vi "GLIMPSE window average.vi"(4 "error in (no error)":errorcluster) -> (0 "error out":errorcluster)   [LabVIEW 2011]
doc: "Performs a (non-destructive) jumping or sliding average of frames in an acquisition file and stores the result in a new acquisition file."
uses:
  Seq file v 1/Offset table.ctl
  Seq file v 1/Offset.ctl
  Seq file v 1/file number.ctl
  GLIMPSE Globals.vi
panel:
  in  "Window type":enum16{"Sliding", "Jumping"}(ring)
  in  "Input from existing":path=path "d:/1.glimpse"
  in  "Output to new directory":path=path "d:/1.glimpse"
  out "Progress":i16(slide) scale=1.0..100.0
  in  "Abort":bool
  in  "Frames to average":u32=8
  in  "Go ahead":bool
  # "This VI does not create header2 data."
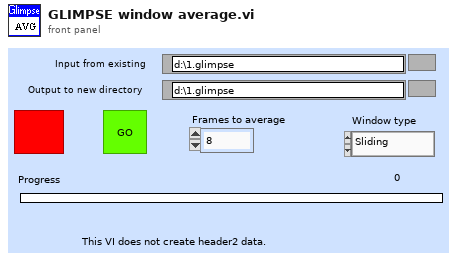
[diagram p1: front panel]
types:
  T1 = typedef "Header2 file data.ctl" = cluster{"Camera":string, "Microscope":string, "Microscope software version":string, "Laser names":string[], "Filter names":string[], "Lasers array":u16[][], "Filter array":u16[], "Flow rate array":dbl[], "Temperature array":dbl[], "Field array":u16[], "Is header2 info present?":bool, "Description Info":string, "Stage xyz array":dbl[][]}
  T2 = typedef "Header file data.ctl" = cluster{"Frames Acquired":u32, "Region width":i32, "Region height":i32, "Element 0 of TTB":u32, "time of 1st frame, \nsec since 1/1/04":dbl, "TTB Array (ms)":u32[], "Offsets Array":T3, "Pixel depth":u32}
  T3 = typedef "Offset table.ctl" = cluster{"offset":T4, "file number":T5}[]
  T4 = typedef "Offset.ctl" = i32
  T5 = typedef "file number.ctl" = u8
  T6 = typedef "Sequence files handle.ctt" = cluster{"Sequence files directory path":path, "Sequence files refnum array":refnum<file>[]}
  T7 = typedef "IMAQ Image.ctl" = refnum<image>
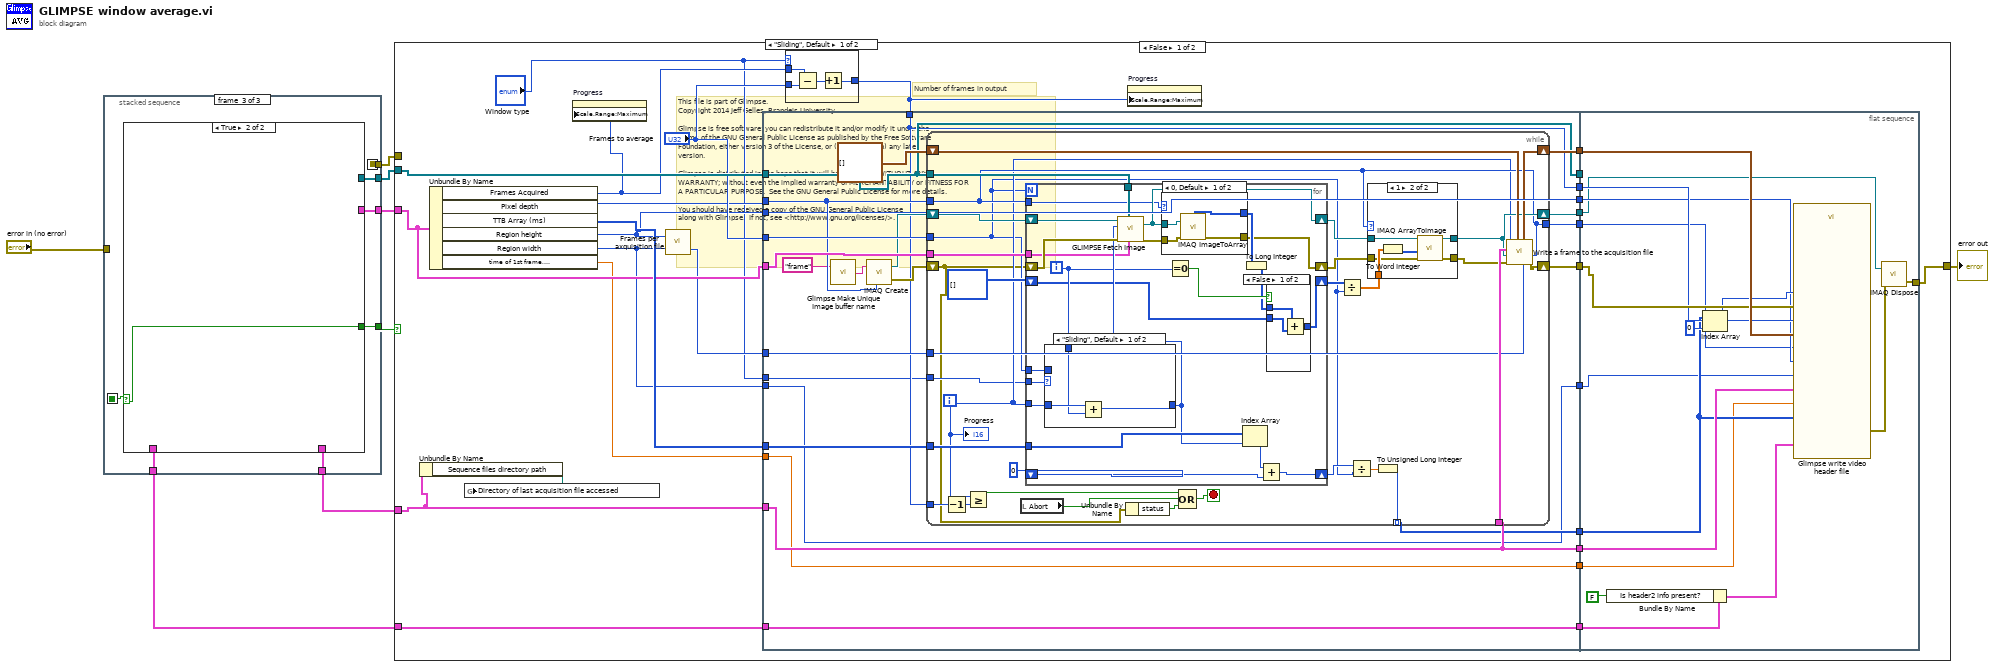
[diagram p0: block diagram]
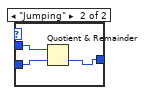
[diagram p2: hidden frame]
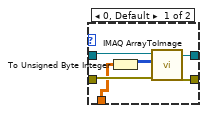
[diagram p3: hidden frame]
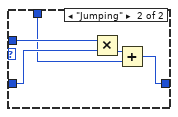
[diagram p4: hidden frame]
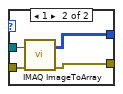
[diagram p6: hidden frame]
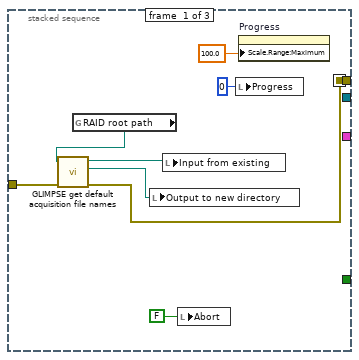
[diagram p8: hidden frame]
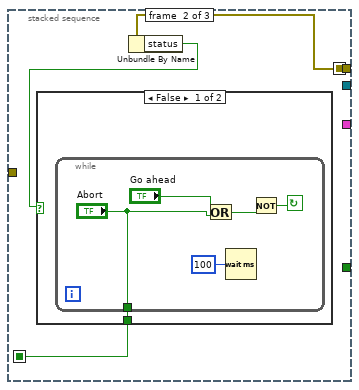
[diagram p9: hidden frame]
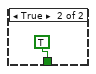
[diagram p10: hidden frame]
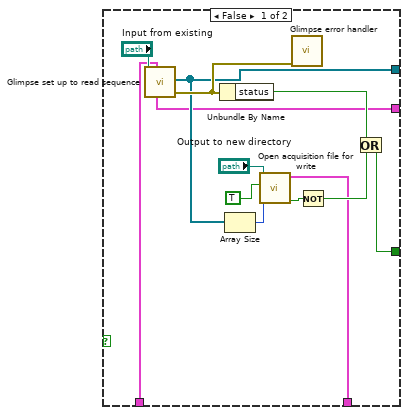
[diagram p11: hidden frame]
diagram:
  # "This file is part of Glimpse. \nCopyright 2014 Jeff Gelles, Brandeis University.    \n\nGlimpse is free software: you can redistribute it and/or modify it under the \nterms of the GNU General Public License as published by the Free Software \nFoundation, either version 3 of the License, or (at your option) any later \nversion.\n\nGlimpse is distributed in the hope that it will be useful, but WITHOUT ANY \nWARRANTY; without even the implied warranty of MERCHANTABILITY or FITNESS FOR \nA PARTICULAR PURPOSE.  See the GNU General Public License for more details.\n\nYou should have received a copy of the GNU General Public License\nalong with Glimpse.  If not, see <http://www.gnu.org/licenses/>."
  n1 = stacked-sequence {
    seq-local: [w11 _ _] -> [_ w19 w29]
    seq-local: [_ w17 _] -> [_ _ w33]
    tunnel: "error in (no error)" -> [w14 _ _]
    tunnel: [_ _ w32] -> w7
    tunnel: [_ _ w31] -> w6
    tunnel: [_ _ w30] -> w5
    tunnel: [_ _ w29] -> w3
    tunnel: [_ _ w28] -> w2
    tunnel: [_ _ w27] -> w1
    frame #0 {
      n2 = global read "GLIMPSE Globals.vi" "RAID root path"() -> (w15:path)
      n3 = call "GLIMPSE get default acquisition file names.vi"("error in"=w14, "RAID root path"=w15) -> ("error out"=w11:errorcluster, "next directory path"=w13:path, "last directory path"=w12:path)  [unwired: 5 out]
      n4 = local write "Output to new directory"(w13) -> ()
      n5 = local write "Input from existing"(w12) -> ()
      n6 = local write "Abort"(FALSE ("Abort")) -> ()
      n7 = local write "Progress"(i16 0 ("Progress")) -> ()
      n8 = property on="Progress" class="Slide (strict)"("Scale.Range:Maximum"=100.0) -> ()  [unwired: 2 in, 2 out]
    }
    frame #1 {
      n9 = Unbundle By Name(w19) -> ("status"=w18:bool)
      n10 = case shown="False" w18 {
        tunnel: [w20 TRUE ("Abort")] -> w17
        frame False {
          n11 = while {
            tunnel: ["Abort"] -> w20
            stop <- w25 continue-if-true
            n12 = Or(x="Go ahead", y="Abort") -> (x .or. y?=w23:bool)
            n13 = Wait (ms)(milliseconds to wait=u32 100) -> ()  [unwired: 1 out]
            n14 = Not(x=w23) -> (.not. x?=w25:bool)
          }
        }
        frame True {
        }
      }
    }
    frame #2 {
      n15 = case shown="True" w33 {
        selector: w33 -> [_ w47]
        tunnel: [w40 w47] -> w32
        tunnel: [w38 _] -> w31
        tunnel: [w36 _] -> w30
        tunnel: [w35 _] -> w28
        tunnel: [w34 _] -> w27
        frame False {
          n16 = call "Glimpse set up to read sequence.vi"("acquisition directory path"="Input from existing") -> ("Header2 file data out"=w34:T1, "Header file data out"=w35:T2, "Acquisition refnum array"=w36:refnum<file>[], "error out"=w39:errorcluster)  [unwired: 1 in, 2 out]
          n17 = Unbundle By Name(w39) -> ("status"=w42:bool)
          n18 = Array Size(array=w36) -> (size(s)=w37:i32)
          n19 = call "Open acquisition file for write.vi"("Number of acquisition files"=w37, "Use new?"=TRUE, "New directory to create"="Output to new directory") -> ("OK?"=w43:bool, "Sequence files handle"=w38:T6)  [unwired: 1 in, 5 out]
          n20 = call "Glimpse error handler.vi"("error in"=w39) -> ()  [unwired: 1 in, 6 out]
          n21 = Not(x=w43) -> (.not. x?=w41:bool)
          n22 = Or(x=w42, y=w41) -> (x .or. y?=w40:bool)
        }
        frame True {
        }
      }
    }
  }
  n23 = case shown="False" w7 {
    tunnel: w6 -> [w51 _]
    tunnel: w5 -> [w75 _]
    tunnel: [w74 w210] -> w4
    tunnel: w3 -> [_ w210]
    tunnel: w2 -> [w69 _]
    tunnel: w1 -> [w49 _]
    frame False {
      # "Number of frames in output"
      n24 = Unbundle By Name(w51) -> ("Sequence files directory path"=w50:path)
      n25 = Unbundle By Name(w69) -> ("Frames Acquired"=w64:u32, "Pixel depth"=w71:u32, "TTB Array (ms)"=w70:u32[], "Region height"=w66:i32, "Region width"=w67:i32, "time of 1st frame, \nsec since 1/1/04"=w65:dbl)
      n26 = global write "GLIMPSE Globals.vi" "Directory of last acquisition file accessed"(w50) -> ()
      n27 = property on="Progress" class="Slide (strict)"("Scale.Range:Maximum"=w64) -> ()  [unwired: 2 in, 2 out]
      n28 = call "Frames per axquisition file.vi"("Output frame width"=w67, "Output frame height"=w66) -> ("Frames per acquisition file"=w68:i32)  [unwired: 1 out]
      n29 = flat-sequence {
        tunnel: "Frames to average" -> [w104]
        tunnel: w51 -> [w100]
        tunnel: [w100] -> w63
        tunnel: w75 -> [w99]
        tunnel: [w99] -> w62
        tunnel: w72 -> [w85]
        tunnel: [w85] -> w61
        tunnel: w71 -> [w94]
        tunnel: w70 -> [w97]
        tunnel: w69 -> [w96]
        tunnel: w68 -> [w95]
        tunnel: w67 -> [w89]
        tunnel: [w89] -> w60
        tunnel: w66 -> [w88]
        tunnel: [w88] -> w59
        tunnel: w65 -> [w87]
        tunnel: [w87] -> w58
        tunnel: [w102] -> w57
        tunnel: [w101] -> w56
        tunnel: [w98] -> w55
        tunnel: [w90] -> w54
        tunnel: [w86] -> w53
        tunnel: "Window type" -> [w84]
        tunnel: w49 -> [w83]
        tunnel: [w83] -> w48
        tunnel: w63 -> [w207]
        tunnel: w62 -> [w205]
        tunnel: [w194] -> w74
        tunnel: w61 -> [w204]
        tunnel: w53 -> [w198]
        tunnel: w60 -> [w200]
        tunnel: w59 -> [w199]
        tunnel: w58 -> [w197]
        tunnel: w57 -> [w208]
        tunnel: w56 -> [w206]
        tunnel: w55 -> [w202]
        tunnel: w54 -> [w196]
        tunnel: w48 -> [w193]
        frame #0 {
          n30 = call "Glimpse Make Unique Image buffer name.vi"("Buffer  base name"="frame" ("Image Name")) -> ("Image Name"=w92:string)  [unwired: 1 out]
          n31 = call "IMAQ Create"("Image Name"=w92, "Image Type"=w94) -> ("New Image"=w93:T7, "error out"=w105:errorcluster)  [unwired: 2 in, 1 out]
          n32 = while {
            tunnel: w104 -> [w108]
            shift-right: [w130] -> w101
            shift-left: w105 -> [w106]
            tunnel: w97 -> [w135]
            tunnel: [w132] -> w98 mode=indexing
            shift-right: [w129] -> w102
            shift-left: T3 [] ("Offset table out") -> [w128]
            tunnel: w100 -> [w127]
            tunnel: w99 -> [w126]
            tunnel: w94 -> [w116]
            tunnel: w96 -> [w125]
            tunnel: w95 -> [w124]
            shift-right: [w117] -> w90
            shift-left: w93 -> [w131]
            tunnel: [w116] -> w86
            tunnel: w85 -> [w113]
            tunnel: w84 -> [w109]
            i -> [w115]
            stop <- w111 stop-if-true
            n33 = Decrement(x=w113) -> (x-1=w114:u32)
            n34 = Greater Or Equal?(x=w115, y=w114) -> (x >= y?=w112:bool)
            n35 = local read "Abort"() -> (w110:bool)
            n36 = for {
              N: w108 -> [_]
              tunnel: w115 -> [w170]
              shift-right: [w154] -> w120
              shift-left: w106 -> [w164]
              shift-right: [w169] -> w134
              shift-left: 0 -> [w168]
              tunnel: w135 -> [w166]
              tunnel: w126 -> [w162]
              tunnel: w125 -> [w161]
              tunnel: w116 -> [w152]
              shift-right: [w153] -> w119
              shift-left: w131 -> [w165]
              shift-right: [w155] -> w122
              shift-left: i32[][] [] -> [w157]
              tunnel: w109 -> [w151]
              tunnel: w108 -> [w150]
              i -> [w158]
              n37 = case shown="\"Sliding\", Default" w151 {
                tunnel: w170 -> [w173 w177]
                tunnel: [w172 w174] -> w163
                tunnel: w158 -> [w171 w175]
                tunnel: w150 -> [_ w178]
                frame "Sliding", Default {
                  n38 = Add(x=w173, y=w171) -> (x+y=w172:i32)
                }
                frame "Jumping" {
                  n39 = Multiply(x=w178, y=w177) -> (x*y=w176:u32)
                  n40 = Add(x=w176, y=w175) -> (x+y=w174:u32)
                }
              }
              n41 = call "GLIMPSE Fetch Image.vi"("Header file data"=w161, "Acqisition files refnums"=w162, "error in"=w164, "Logical Frame Number\n(starting with zero)"=w163, "Image In"=w165) -> ("error out"=w160:errorcluster, "Image Out"=w153:T7)  [unwired: 2 in, 3 out]
              n42 = case shown="0, Default" w152 {
                tunnel: w153 -> [w185 w190]
                tunnel: w160 -> [w186 w189]
                tunnel: [w183 w187] -> w156
                tunnel: [w184 w188] -> w154
                frame 0, Default {
                  n43 = call "IMAQ ImageToArray"("error in (no error)"=w186, "Image"=w185) -> ("error out"=w184:errorcluster, "Image Pixels (U8)"=w183:u8[][])  [unwired: 1 in, 4 out]
                }
                frame 1 {
                  n44 = call "IMAQ ImageToArray"("error in (no error)"=w189, "Image"=w190) -> ("error out"=w188:errorcluster, "Image Pixels (I16)"=w187:i16[][])  [unwired: 1 in, 4 out]
                }
              }
              n45 = Equal To 0?(x=w158) -> (x = 0?=w159:bool)
              n46 = Index Array(array=w166, index=w163) -> (element=w167:u32)
              n47 = To Long Integer(number=w156) -> (32bit integer=w149:i32[][])
              n48 = Add(x=w167, y=w168) -> (x+y=w169:u32)
              n49 = case shown="False" w159 {
                tunnel: w157 -> [w180 _]
                tunnel: [w179 w182] -> w155
                tunnel: w149 -> [w181 w182]
                frame False {
                  n50 = Add(x=w181, y=w180) -> (x+y=w179:i32[][])
                }
                frame True {
                }
              }
            }
            n51 = Unbundle By Name(w106) -> ("status"=w107:bool)
            n52 = Compound Arithmetic op=OR(w112, w110, w107) -> (w111:bool)
            n53 = Divide(x=w122, y=w108) -> (x/y=w121:dbl[][])
            n54 = Divide(x=w134, y=w108) -> (x/y=w133:dbl)
            n55 = case shown="1" w116 {
              tunnel: w121 -> [w137 w147]
              tunnel: w120 -> [w139 w146]
              tunnel: w119 -> [w140 w145]
              tunnel: [w141 w144] -> w117
              tunnel: [w142 w143] -> w118
              frame 0, Default {
                n56 = To Unsigned Byte Integer(number=w137) -> (unsigned 8bit integer=w138:u8[][])
                n57 = call "IMAQ ArrayToImage"("error in (no error)"=w139, "Image Pixels (U8)"=w138, "Image"=w140) -> ("error out"=w142:errorcluster, "Image Out"=w141:T7)  [unwired: 3 in, 4 out]
              }
              frame 1 {
                n58 = To Word Integer(number=w147) -> (16bit integer=w148:i16[][])
                n59 = call "IMAQ ArrayToImage"("error in (no error)"=w146, "Image Pixels (I16)"=w148, "Image"=w145) -> ("error out"=w143:errorcluster, "Image Out"=w144:T7)  [unwired: 3 in, 4 out]
              }
            }
            n60 = To Unsigned Long Integer(number=w133) -> (unsigned 32bit integer=w132:u32)
            n61 = call "Write a frame to the acquisition file.vi"("Pixel depth"=w116, "Frames per acquisition file"=w124, "Offset table in"=w128, "error in"=w118, "Image In"=w117, "Sequence files handle"=w127, "Last frame number written in"=w115) -> ("error out"=w130:errorcluster, "Offset table out"=w129:T3)  [unwired: 3 out]
            "Progress" <- w115
          }
        }
        frame #1 {
          n62 = for {
            tunnel: w205 -> [w209] mode=indexing
            n63 = Close File(refnum=w209) -> ()  [unwired: 1 in, 2 out]
          }
          n64 = Bundle By Name(cluster=w193, "Is header2 info present?"=FALSE) -> (w191:T1)
          n65 = Index Array(array=w202, index=0 ("Index")) -> (element=w201:u32)
          n66 = call "Glimpse write video header file.vi"("Number of frames"=w204, "Sequence files handle"=w207, "Pixel depth\n(0=8 bit; 1= 16 bit)"=w198, "error in"=w206, "TTB Array"=w202, "Offsets Array"=w208, "Header2 file data"=w191, "Region width"=w200, "Region height"=w199, "Element 0 of TTB"=w201, "time of 1st frame, \nsec since 1/1/04"=w197) -> ("error out"=w195:errorcluster)  [unwired: 8 in]
          n67 = call "IMAQ Dispose"("Image"=w196, "error in (no error)"=w195) -> ("error out"=w194:errorcluster)  [unwired: 1 in, 3 out]
        }
      }
      n68 = case shown="\"Sliding\", Default" "Window type" {
        tunnel: "Frames to average" -> [w78 w81]
        tunnel: [w77 w80] -> w72
        tunnel: w64 -> [w76 w82]
        frame "Sliding", Default {
          n69 = Subtract(x=w76, y=w78) -> (x-y=w79:u32)
          n70 = Increment(x=w79) -> (x+1=w77:u32)
        }
        frame "Jumping" {
          n71 = Quotient & Remainder(x=w82, y=w81) -> (floor(x/y)=w80:u32)  [unwired: 1 out]
        }
      }
      n72 = property on="Progress" class="Slide (strict)"("Scale.Range:Maximum"=w72) -> ()  [unwired: 2 in, 2 out]
    }
    frame True {
    }
  }
  "error out" <- w4
